vi "Constant Curvature Drive.vi"(6 "Auxilery?":bool, 8 "Turbo?":bool, 9 "QuickTurn?":bool, 10 "Speed":dbl(slide)=0.047244094488188976 scale=-1.0..1.0, 11 "Curve":dbl(slide)=0.07874015748031496 scale=-1.0..1.0) -> (0 "Right Percent Setpoint":dbl, 3 "Left Percent Setpoint":dbl)   [LabVIEW 2018]
uses:
  <vilib>/Rock Robotics/WPI/Joystick/WPI_JoystickRatioCurveMapping.vi
panel:
  in  "Auxilery Max %Output":dbl=0.25
  in  "Turbo Max %Output":dbl=0.9
  in  "Deadband":dbl=0.08
  in  "Sensitivity":dbl=0.1
  in  "Normal Max %Output":dbl=0.7
  # "Drive like a car, where any turning input will yield the same curve, regardless of the speed it is traveled at\nUse Velocity PIDF with these outputs, it fights turning over shoot and makes you drive straight\n1718 said to do these things but 4810 put it into code"
  # "Auxilery is like if something is too high"
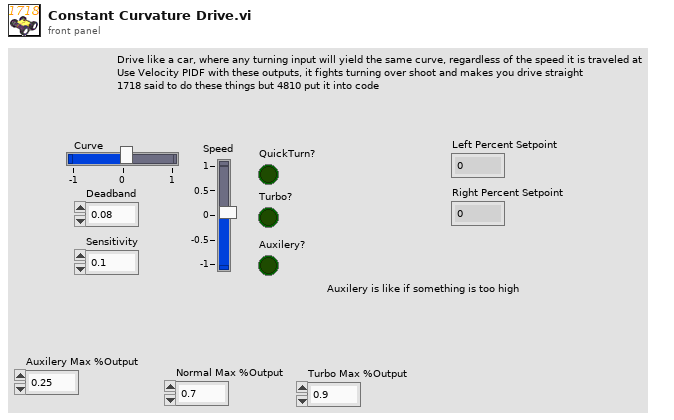
[diagram p1: front panel]
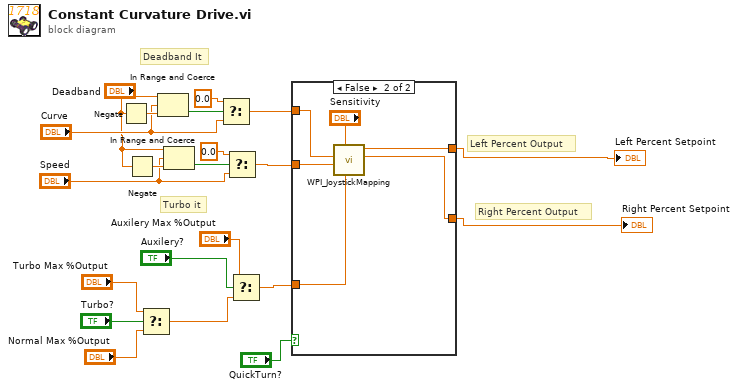
[diagram p0: block diagram]
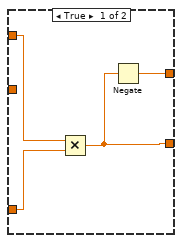
[diagram p2: hidden frame]
diagram:
  # "Right Percent Output"
  # "Left Percent Output"
  # "Turbo it"
  # "Deadband It"
  n1 = Negate(x="Deadband") -> (-x=w19:dbl)
  n2 = Negate(x="Deadband") -> (-x=w17:dbl)
  n3 = Select(t="Turbo Max %Output", s="Turbo?", f="Normal Max %Output") -> (s? t:f=w1:dbl)
  n4 = In Range and Coerce(upper limit="Deadband", x="Curve", lower limit=w19) -> (In Range?=w21:bool)  [unwired: 1 out]
  n5 = In Range and Coerce(upper limit="Deadband", x="Speed", lower limit=w17) -> (In Range?=w15:bool)  [unwired: 1 out]
  n6 = Select(t=0.0 ("Default Value"), s=w21, f="Curve") -> (s? t:f=w12:dbl)
  n7 = Select(t=0.0 ("Default Value"), s=w15, f="Speed") -> (s? t:f=w11:dbl)
  n8 = Select(t="Auxilery Max %Output", s="Auxilery?", f=w1) -> (s? t:f=w4:dbl)
  n9 = case shown="False" "QuickTurn?" {
    tunnel: w12 -> [w25 w31]
    tunnel: w11 -> [_ w30]
    tunnel: w4 -> [w24 w28]
    tunnel: [w22 w27] -> w6
    tunnel: [w23 w26] -> w5
    frame True {
      n10 = Multiply(x=w25, y=w24) -> (x*y=w23:dbl)
      n11 = Negate(x=w23) -> (-x=w22:dbl)
    }
    frame False {
      n12 = call-poly <vilib>:"WPI_JoystickMapping.vi"("Max Output"=w28, "Sensitivity"="Sensitivity", "Y axis value (Speed)"=w30, "X axis value (Curve)"=w31) -> ("Right Motor Value"=w26:dbl, "Left Motor Value"=w27:dbl)  [unwired: 6 in]
    }
  }
  "Left Percent Setpoint" <- w6
  "Right Percent Setpoint" <- w5
